vi "wristAngleToEncoderCounts.vi"(1 "wristAngle":dbl) -> (0 "wristEncoderCounts":dbl)   [LabVIEW 2020]
panel:
  in  "b":dbl=4.21467
  in  "m":dbl=0.52936
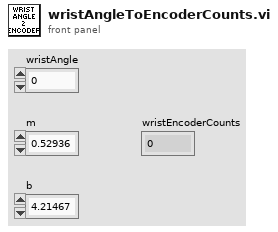
[diagram p1: front panel]
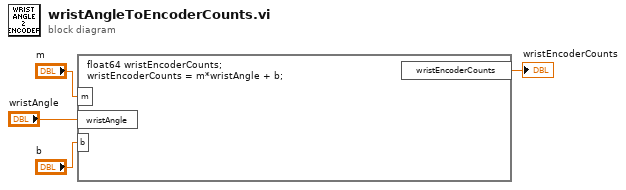
[diagram p0: block diagram]
diagram:
  n1 = formula code="float64 wristEncoderCounts;\nwristEncoderCounts = m*wristAngle + b;"("m"="m", "wristAngle"="wristAngle", "b"="b") -> ("wristEncoderCounts"=→"wristEncoderCounts":dbl)
